vi "Build getReading XML.vi"(8 "error in (no error)":errorcluster, 11 "Device":string="d:outtmp") -> (0 "error out":errorcluster, 3 "XML":string)   [LabVIEW 2013]
uses:
  Add Child to Document.vi
  Add Child to Element.vi
  Add Text to Element.vi
  <vilib>/xml/Close Reference(Node).vi
  <vilib>/xml/NI_XML.lvlib
  <resource>/objmgr/DOMUserDefRef.rc
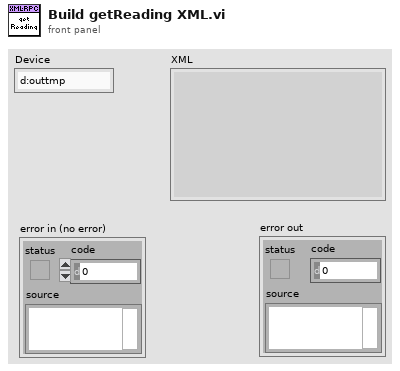
[diagram p1: front panel]
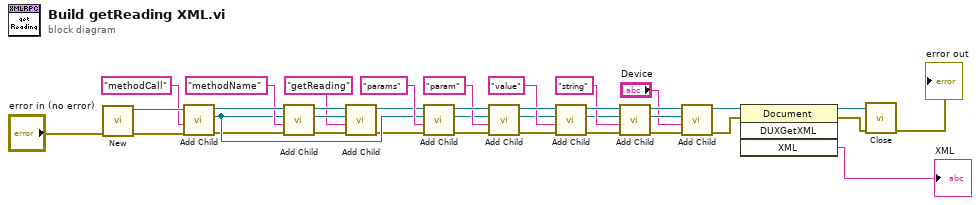
[diagram p0: block diagram]
diagram:
  n1 = call <vilib>:"New.vi"("error in (no error)"="error in (no error)") -> ("error out"=w10:errorcluster, "DOM document out"=w37:refnum<k20>)  [unwired: 7 in]
  n2 = call-poly "Add Child.vi"("error in (no error)"=w10, "Tag Name"="methodCall", "DOM document"=w37) -> ("error out"=w9:errorcluster, "Child Element"=w16:refnum<k20>, "DOM document out"=w35:refnum<k20>)  [unwired: 6 in]
  n3 = call-poly "Add Child.vi"("error in (no error)"=w9, "Tag Name"="methodName", "Parent Element"=w16, "DOM document"=w35) -> ("error out"=w8:errorcluster, "Child Element"=w22:refnum<k20>, "DOM document out"=w23:refnum<k20>)  [unwired: 5 in]
  n4 = call-poly "Add Child.vi"("error in (no error)"=w8, "Text"="getReading" ("Node Value"), "Parent Element"=w22, "DOM document"=w23) -> ("error out"=w7:errorcluster, "DOM document out"=w17:refnum<k20>)  [unwired: 5 in, 1 out]
  n5 = call-poly "Add Child.vi"("error in (no error)"=w7, "Tag Name"="params", "Parent Element"=w16, "DOM document"=w17) -> ("error out"=w6:errorcluster, "Child Element"=w30:refnum<k20>, "DOM document out"=w32:refnum<k20>)  [unwired: 5 in]
  n6 = call-poly "Add Child.vi"("error in (no error)"=w6, "Tag Name"="param", "Parent Element"=w30, "DOM document"=w32) -> ("error out"=w5:errorcluster, "Child Element"=w25:refnum<k20>, "DOM document out"=w29:refnum<k20>)  [unwired: 5 in]
  n7 = call-poly "Add Child.vi"("error in (no error)"=w5, "Tag Name"="value", "Parent Element"=w25, "DOM document"=w29) -> ("error out"=w4:errorcluster, "Child Element"=w24:refnum<k20>, "DOM document out"=w28:refnum<k20>)  [unwired: 5 in]
  n8 = call-poly "Add Child.vi"("error in (no error)"=w4, "Tag Name"="string", "Parent Element"=w24, "DOM document"=w28) -> ("error out"=w3:errorcluster, "Child Element"=w19:refnum<k20>, "DOM document out"=w20:refnum<k20>)  [unwired: 5 in]
  n9 = call-poly "Add Child.vi"("error in (no error)"=w3, "Text"="Device", "Parent Element"=w19, "DOM document"=w20) -> ("error out"=w13:errorcluster, "DOM document out"=w14:refnum<k20>)  [unwired: 5 in, 1 out]
  n10 = invoke class="Document" method="DUXGetXML"(reference=w14, error in=w13) -> (reference out=w15:refnum<k20>, error out=w12:errorcluster, "XML"=→"XML":string)  [unwired: 2 in, 1 out]
  n11 = call-poly <vilib>:"Close.vi"("error in (no error)"=w12, "node"=w15) -> ("error out"=→"error out":errorcluster)  [unwired: 7 in]
